vi "Hellevator 2 Electric Boogaloo.vi"() -> (2 "Position (Raw Sensor Units)":i32)   [LabVIEW 2017]
uses:
  <vilib>/Rock Robotics/WPI/ThirdParty/Phoenix-LabVIEW/Motor Controller/Controls/CTRE_Phoenix_MotorControl_ControlMode.ctl
  <vilib>/Rock Robotics/WPI/Utilities/WPI_GetSetVariantRefNum.vi
  Robot Global Data.vi
  <vilib>/Rock Robotics/WPI/ThirdParty/Phoenix-LabVIEW/Motor Controller/Get/CTRE_Phoenix_MotorController_GetPulseWidthAll.vi
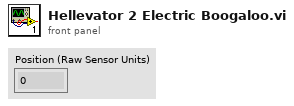
[diagram p1: front panel]
types:
  T1 = typedef "WPI_MotorControlDeviceRef.ctl" = cluster{"DeviceStatus":errorcluster, "Type":T2, "PWM":cluster{"PWM Channel":T3, "DeadBand":T4}, "CAN":cluster{"Device Number":u8, "SetOutput VI Ref":variant, "GetOutput VI Ref":variant, "Enable VI Ref":variant, "Disable VI Ref":variant, "Data":variant}, "Invert":bool, "DIO PWM":cluster{"PWM \"Enable\" Channel":T3, "DIOChannel":T5, "PWM Rate":dbl}}
  T2 = typedef "WPI_MotorControlType.ctl" = enum16{"PWM", "CAN", "DIO PWM"}
  T3 = typedef "FPGA_DIOPWMChannel.ctl" = enum8{"PWM 0", "PWM 1", "PWM 2", "PWM 3", "PWM 4", "PWM 5", "PWM 6", "PWM 7", "PWM 8", "PWM 9", "PWM MXP 0", "PWM MXP 1", "PWM MXP 2", "PWM MXP 3", "PWM MXP 4", "PWM MXP 5", "PWM MXP 6", "PWM MXP 7", "PWM MXP 8", "PWM MXP 9", "Invalid"}
  T4 = typedef "WPI_PWMDeadband.ctl" = cluster{"Name":string, "maxPositivePwm":i32, "minPositivePwm":i32, "centerPwm":i32, "maxNegativePwm":i32, "minNegativePwm":i32, "angularRange":u16}
  T5 = typedef "FPGA_DIOChannel.ctl" = enum8{"DIO 0", "DIO 1", "DIO 2", "DIO 3", "DIO 4", "DIO 5", "DIO 6", "DIO 7", "DIO 8", "DIO 9", "DIO MXP 0", "DIO MXP 1", "DIO MXP 2", "DIO MXP 3", "DIO MXP 4", "DIO MXP 5", "DIO MXP 6", "DIO MXP 7", "DIO MXP 8", "DIO MXP 9", "DIO MXP 10", "DIO MXP 11", "DIO MXP 12", "DIO MXP 13", "DIO MXP 14", "DIO MXP 15", "SPI Port CS1", "SPI Port CS2", "SPI Port CS3", "SPI Port MISO", "SPI Port MOSI", "Invalid"}
  T6 = typedef "WPI_JoystickDevRef.ctl" = cluster{"Device":T7}
  T7 = typedef "WPI_JoystickDeviceEnum.ctl" = enum16{"USB 0", "USB 1", "USB 2", "USB 3", "USB 4", "USB 5"}
  T8 = typedef "CTRE_Phoenix_MotorControl_ControlMode.ctl" = u16
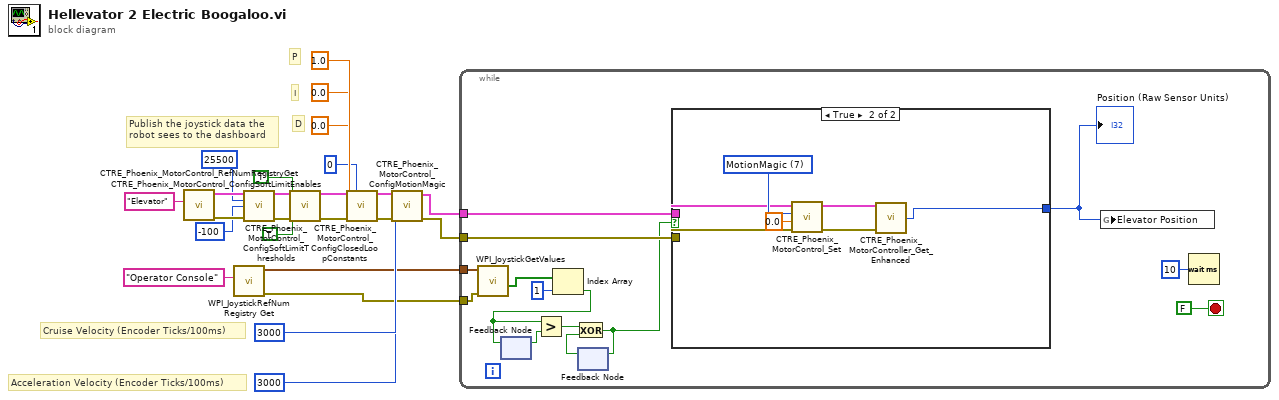
[diagram p0: block diagram]
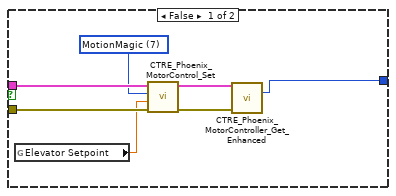
[diagram p2: hidden frame]
diagram:
  # "D"
  # "I"
  # "P"
  # "Acceleration Velocity (Encoder Ticks/100ms)"
  # "Cruise Velocity (Encoder Ticks/100ms)"
  # "Publish the joystick data the\nrobot sees to the dashboard"
  n1 = call <vilib>:"CTRE_Phoenix_MotorControl_RefNumRegistryGet.vi"("refnum name"="Elevator") -> ("error out"=w22:errorcluster, "PhoenixMotorControlDevRef"=w23:T1)  [unwired: 9 in]
  n2 = call <vilib>:"WPI_JoystickRefNum Registry Get.vi"("refnum name"="Operator Console") -> ("error out"=w2:errorcluster, "JoystickDevRef"=w1:T6)  [unwired: 9 in]
  n3 = call <vilib>:"CTRE_Phoenix_MotorControl_ConfigSoftLimitThresholds.vi"("PhoenixMotorControlDevRef"=w23, "Forward Soft Limit"=25500, "Reverse Soft Limit"=-100, "error in (no error)"=w22) -> ("PhoenixMotorControlDevRef"=w19:T1, "error out"=w18:errorcluster)  [unwired: 10 in]
  n4 = call <vilib>:"CTRE_Phoenix_MotorControl_ConfigSoftLimitEnables.vi"("PhoenixMotorControlDevRef"=w19, "Forward Soft Limit Enable"=TRUE, "Reverse Soft Limit Enable"=TRUE, "error in (no error)"=w18) -> ("PhoenixMotorControlDevRef"=w15:T1, "error out"=w14:errorcluster)  [unwired: 10 in]
  n5 = call <vilib>:"CTRE_Phoenix_MotorControl_ConfigClosedLoopConstants.vi"("PhoenixMotorControlDevRef"=w15, "slotIdx"=0, "P"=1.0, "I"=0.0, "D"=0.0, "error in (no error)"=w14) -> ("PhoenixMotorControlDevRef"=w9:T1, "error out"=w8:errorcluster)  [unwired: 8 in]
  n6 = call <vilib>:"CTRE_Phoenix_MotorControl_ConfigMotionMagic.vi"("error in (no error)"=w8, "Acceleration"=3000, "Cruise Velocity"=3000, "PhoenixMotorControlDevRef"=w9) -> ("error out"=w6:errorcluster, "PhoenixMotorControlDevRef"=w7:T1)  [unwired: 6 in]
  n7 = while {
    tunnel: w7 -> [w36]
    tunnel: w6 -> [w35]
    tunnel: w2 -> [w31]
    tunnel: w1 -> [w30]
    stop <- FALSE stop-if-true
    n8 = call <vilib>:"WPI_JoystickGetValues.vi"("error in (no error)"=w31, "JoystickDevRef"=w30) -> ("Buttons"=w33:bool[])  [unwired: 5 in, 4 out]
    n9 = feedback #1() -> (w29:bool)  [unwired: 1 in]
    n10 = Index Array(array=w33, index=1) -> (element=w26:bool)
    n11 = feedback-in #1(w26) -> ()
    n12 = Greater?(x=w26, y=w29) -> (0:w28:bool)
    n13 = feedback #2() -> (w27:bool)  [unwired: 1 in]
    n14 = Exclusive Or(1:w27, 2:w28) -> (0:w25:bool)
    n15 = feedback-in #2(w25) -> ()
    n16 = case shown="True" w25 {
      tunnel: w36 -> [w45 w49]
      tunnel: w35 -> [w44 w48]
      tunnel: [w43 w46] -> w34
      frame False {
        w42 = T8 7 items=["PercentOutput"=0, "Position"=1, "Velocity"=2, "Current"=3, "Follower"=5, "MotionProfile"=6, "MotionMagic"=7, "MotionMagicArc"=8, "MotionProfileArc"=10, "Disabled"=15] ("Control Mode")
        n17 = global read "Robot Global Data.vi" "Elevator Setpoint"() -> (w39:dbl)
        n18 = call <vilib>:"CTRE_Phoenix_MotorControl_Set.vi"("error in (no error)"=w44, "Output"=w39, "Control Mode"=w42, "PhoenixMotorControlDevRef"=w45) -> ("error out"=w40:errorcluster, "PhoenixMotorControlDevRef"=w41:T1)  [unwired: 6 in]
        n19 = call-poly <vilib>:"CTRE_Phoenix_MotorController_Get_Enhanced.vi"("PhoenixMotorControlDevRef"=w41, "error in"=w40) -> ("Pulse Width Position"=w43:i32)  [unwired: 8 in, 5 out]
      }
      frame True {
        w50 = T8 7 items=["PercentOutput"=0, "Position"=1, "Velocity"=2, "Current"=3, "Follower"=5, "MotionProfile"=6, "MotionMagic"=7, "MotionMagicArc"=8, "MotionProfileArc"=10, "Disabled"=15] ("Control Mode")
        n20 = call <vilib>:"CTRE_Phoenix_MotorControl_Set.vi"("error in (no error)"=w48, "Output"=0.0, "Control Mode"=w50, "PhoenixMotorControlDevRef"=w49) -> ("error out"=w51:errorcluster, "PhoenixMotorControlDevRef"=w52:T1)  [unwired: 6 in]
        n21 = call-poly <vilib>:"CTRE_Phoenix_MotorController_Get_Enhanced.vi"("PhoenixMotorControlDevRef"=w52, "error in"=w51) -> ("Pulse Width Velocity"=w46:i32)  [unwired: 8 in, 5 out]
      }
    }
    "Position (Raw Sensor Units)" <- w34
    n22 = global write "Robot Global Data.vi" "Elevator Position"(w34) -> ()
    n23 = Wait (ms)(milliseconds to wait=u32 10) -> ()  [unwired: 1 out]
  }
